vi "GetActivePortNames.vi"(0 "Matched Configurations In":T3(array[cluster]) {"Static Drive Configuration"."Indexer Mode  (FSA)" items=["Incremental", "Absolute"]; "Static Drive Configuration"."Buffer at Stop (SSH)" items=["Clear buffer", "Save and Continue"]; "Static Drive Configuration"."Buffer at Limit (SSG)" items=["Clear buffer", "Save and Continue"]; "Static Drive Configuration"."RS232 Echo Control (SSA)" items=["Echo ON", "Echo OFF"]; "Static Drive Configuration"."Reference edge of Home (OSH)" items=["CW", "CCW"]; "Static Drive Configuration"."Encoder Z for Home (OSD)" items=["Don't use", "Enable"]; "Static Drive Configuration"."Home Switch Sense (OSC)" items=["Normally Open", "Normally Closed"]; "Static Drive Configuration"."Home Position (OSB)" items=["Anywhere in Switch", "Edge of Switch"]; "Static Drive Configuration"."Limit Switch Sense (OSA)" items=["Normally Closed", "Normally Open"]; "Static Drive Configuration"."Limit Disable (LD)" items=["Both Enabled", "CW Disabled", "CCW Disabled", "Both Disabled"]; "Static Drive Configuration"."Stall Detect (FSH)" items=["Disable", "Enable"]; "Static Drive Configuration"."OP2 in Deadband (FSG)" items=["Don't Use", "ACTIVATE"]; "Static Drive Configuration"."Stop on Trigger 3 (FSF)" items=["Ignore", "STOP!"]; "Static Drive Configuration"."Activate OP1 on stall (FSE)" items=["Do not Activate", "ACTIVATE!"]; "Static Drive Configuration"."Stop on Stall (FSD)" items=["Continue", "STOP"]; "Static Drive Configuration"."Position Maintenance (FSC)" items=["Disabled", "Enabled"]; "Static Drive Configuration"."Step Mode  (FSB)" items=["Motor", "Encoder"]; "Static Drive Configuration"."Encoder Resolution (ER)" min=1 max=50000; "Static Drive Configuration"."Dead Band Window (DW)" min=0 max=999999999; "Static Drive Configuration"."Dead Band (DB)" min=0 max=999999999; "Static Drive Configuration"."Correction Gain % (CG)" items=["n/a", "12.5", "25", "37.5", "50", "62.5", "75", "87.5", "100"]; "Channel Properties"."Current Pos" format="%.2f"; "Channel Properties"."Backlash/Eng units" format="%.2f"; "Channel Properties"."Pulses/rev" format="%.2f"; "Channel Properties"."Pos Tolerance" format="%.2f"; "Channel Properties"."Pulses/unit" format="%.2f"; "Channel Properties"."Acc. Min" format="%.2f"; "Channel Properties"."Acc. Max" format="%.2f"; "Channel Properties"."Vel. Min" format="%.2f"; "Channel Properties"."Vel. Max" format="%.2f"; "Channel Properties"."Acc. Default" format="%.2f"; "Channel Properties"."Vel. Default" format="%.2f"}) -> (1 "Port Name Array":string[](array[string]), 2 "Drive Type Array":string[](array[string]))   [LabVIEW 2010]
uses:
  DriveProperties.ctl
  DriveStaticConfig.ctl
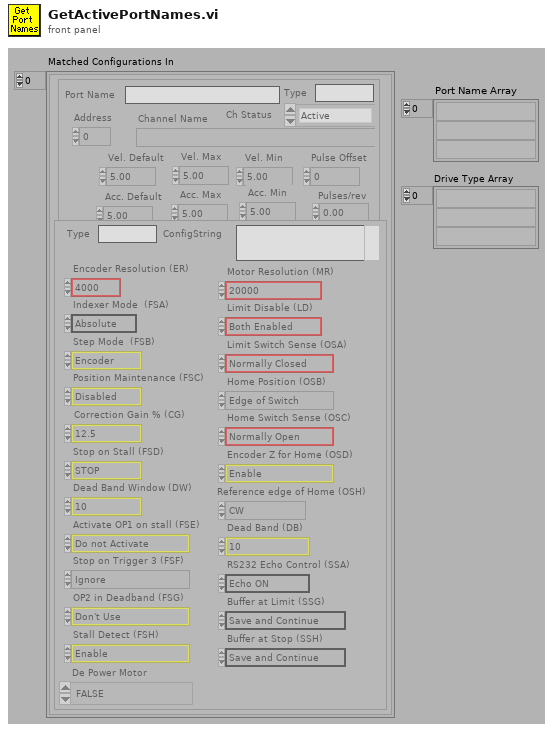
[diagram p1: front panel]
types:
  T1 = typedef "DriveProperties.ctl" = cluster{"Channel Name":string, "Vel. Default":dbl, "Acc. Default":dbl, "Vel. Max":dbl, "Vel. Min":dbl, "Acc. Max":dbl, "Acc. Min":dbl, "Pulses/unit":dbl, "Address":u8, "Pulse Offset":i32, "Pos Tolerance":dbl, "Pulses/rev":dbl, "Backlash/Eng units":dbl, "Current Pos":dbl, "Ch Status":enum16{"Active", "Offline", "Simulate"}, "Port Name":string, "Axis Transform mode":string, "Metadata Ch Name":string, "Type":string}
  T2 = typedef "DriveStaticConfig.ctl" = cluster{"Correction Gain % (CG)":u16, "Dead Band (DB)":i32, "Dead Band Window (DW)":i32, "Encoder Resolution (ER)":i32, "Step Mode  (FSB)":u16, "Position Maintenance (FSC)":u16, "Stop on Stall (FSD)":u16, "Activate OP1 on stall (FSE)":u16, "Stop on Trigger 3 (FSF)":u16, "OP2 in Deadband (FSG)":u16, "Stall Detect (FSH)":u16, "Limit Disable (LD)":u16, "Motor Resolution (MR)":enum16{"200", "400", "1000", "2000", "4000", "5000", "10000", "12800", "18000", "20000", "21600", "25000", "25400", "25600", "36000", "50000", "278528", "425984", "507904", "614400", "655360", "819200", "1024000"}, "Limit Switch Sense (OSA)":u16, "Home Position (OSB)":u16, "Home Switch Sense (OSC)":u16, "Encoder Z for Home (OSD)":u16, "Reference edge of Home (OSH)":u16, "RS232 Echo Control (SSA)":u16, "Buffer at Limit (SSG)":u16, "Buffer at Stop (SSH)":u16, "Indexer Mode  (FSA)":u16, "Type":string, "ConfigString":string, "De Power Motor":enum16{"TRUE", "FALSE"}}
  T3 = cluster{"Channel Properties":T1, "Static Drive Configuration":T2}[]
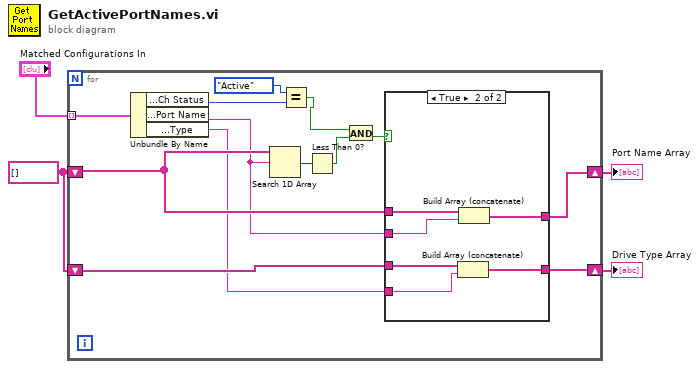
[diagram p0: block diagram]
diagram:
  w2 = string[] []
  n1 = for {
    tunnel: "Matched Configurations In" -> [w17] mode=indexing
    shift-right: [w13] -> w3
    shift-left: w2 -> [w15]
    shift-right: [w6] -> w1
    shift-left: w2 -> [w7]
    n2 = Unbundle By Name(w17) -> ("Channel Properties.Ch Status"=w9:enum16{"Active", "Offline", "Simulate"}, "Channel Properties.Port Name"=w14:string, "Static Drive Configuration.Type"=w5:string)
    n3 = Search 1D Array(1D array=w15, element=w14) -> (index of element=w16:i32)  [unwired: 1 out]
    n4 = Equal?(x=enum16{"Active", "Offline", "Simulate"}."Active" ("Channel Properties.Ch Status"), y=w9) -> (x = y?=w8:bool)
    n5 = Less Than 0?(x=w16) -> (x < 0?=w12:bool)
    n6 = And(x=w8, y=w12) -> (x .and. y?=w11:bool)
    n7 = case shown="True" w11 {
      tunnel: w15 -> [w19 w25]
      tunnel: w14 -> [_ w24]
      tunnel: [w19 w23] -> w13
      tunnel: w7 -> [w18 w22]
      tunnel: [w18 w21] -> w6
      tunnel: w5 -> [_ w20]
      frame False {
      }
      frame True {
        n8 = Build Array (concatenate)(w22, w20) -> (w21:string[])
        n9 = Build Array (concatenate)(w25, w24) -> (w23:string[])
      }
    }
  }
  "Port Name Array" <- w3
  "Drive Type Array" <- w1
